vi "Select Measurement.vi"(0 "Meas Type":T1, 11 "Error In":errorcluster) -> (4 "Y axis commands>>>":string[](array[string]), 6 "X axix commands>>>":string[](array[string]), 15 "Error Out":errorcluster)   [LabVIEW 2013]
uses:
  Controls/Meas Type.ctl
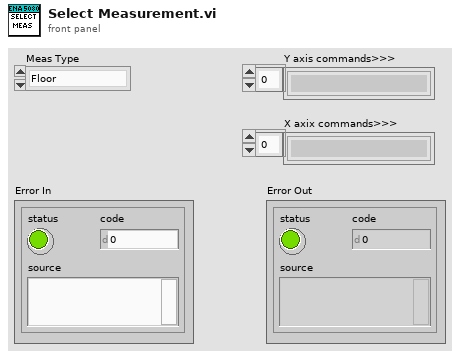
[diagram p1: front panel]
types:
  T1 = typedef "Meas Type.ctl" = enum16{"Floor", "Roof", "Buckling", "Charge Transfer"}
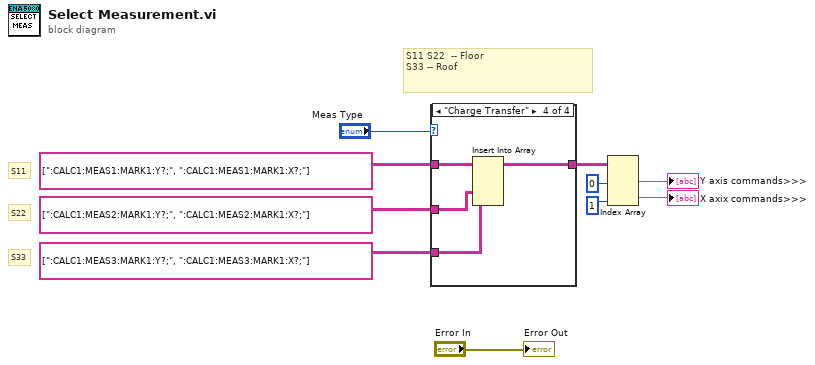
[diagram p0: block diagram]
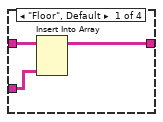
[diagram p2: hidden frame]
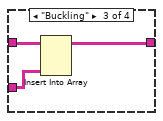
[diagram p4: hidden frame]
diagram:
  # "S11 S22  -- Floor\nS33 -- Roof"
  # "S33"
  # "S22"
  # "S11"
  n1 = case shown="\"Charge Transfer\"" "Meas Type" {
    tunnel: string[][] [[":CALC1:MEAS1:MARK1:Y?;", ":CALC1:MEAS1:MARK1:X?;"]] -> [w13 _ w17 w21]
    tunnel: string[][] [[":CALC1:MEAS2:MARK1:Y?;", ":CALC1:MEAS2:MARK1:X?;"]] -> [w12 _ w16 w20]
    tunnel: string[][] [[":CALC1:MEAS3:MARK1:Y?;", ":CALC1:MEAS3:MARK1:X?;"]] -> [_ w14 _ w19]
    tunnel: [w11 w14 w15 w18] -> w6
    frame "Floor", Default {
      n2 = Insert Into Array(array=w13, new element=w12) -> (w11:string[][])  [unwired: 2 in]
    }
    frame "Roof" {
    }
    frame "Buckling" {
      n3 = Insert Into Array(array=w17, new element=w16) -> (w15:string[][])  [unwired: 2 in]
    }
    frame "Charge Transfer" {
      n4 = Insert Into Array(array=w21, new element #1=w20, new element #2=w19) -> (w18:string[][])  [unwired: 2 in]
    }
  }
  n5 = Index Array(array=w6, index (col) #1=0 ("disabled index (col)"), index (col) #2=1 ("index (col)")) -> (element #1=→"Y axis commands>>>":string[], element #2=→"X axix commands>>>":string[])  [unwired: 2 in]
  "Error Out" <- "Error In"
